vi "Conn Get Properties.vi"(4 "error in (no error)":errorcluster, 7 "connection reference":T2) -> (0 "error out":errorcluster, 1 "connection properties":T1, 3 "connection reference out":T2)   [LabVIEW 2017, in "NI_Database_API.lvlib"]
doc: "Gets properties of the object as determined by the inputs. This VI works for connections, commands, recordsets, columns, and parameters. Wire data to the reference input to determine the polymorphic instance to use or manually select the instance."
uses:
  <vilib>/addons/database/NI_Database_API.lvlib
  <vilib>/addons/database/Connection.llb/Conn ObjectReference.ctl
  <vilib>/addons/database/Connection.llb/Conn Properties.ctl
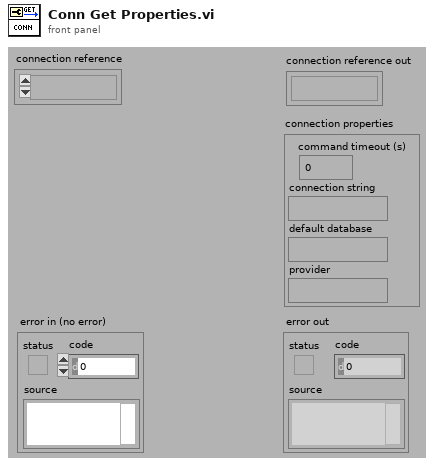
[diagram p1: front panel]
types:
  T1 = typedef "NI_Database_API.lvlib/Conn Properties.ctl" = cluster{"command timeout (s)":i32, "connection string":string, "default database":string, "provider":string}
  T2 = typedef "NI_Database_API.lvlib/Conn ObjectReference.ctl" = refnum<k1>
  T3 = typedef "NI_Database_API.lvlib/Conn DataMembers.ctl" = cluster{"ADODB._Connection":refnum<k7>, "recordset objects":i32, "command objects":i32}
  T4 = cluster{"CommandTimeout":i32, "ConnectionString":string, "DefaultDatabase":string, "Provider":string}
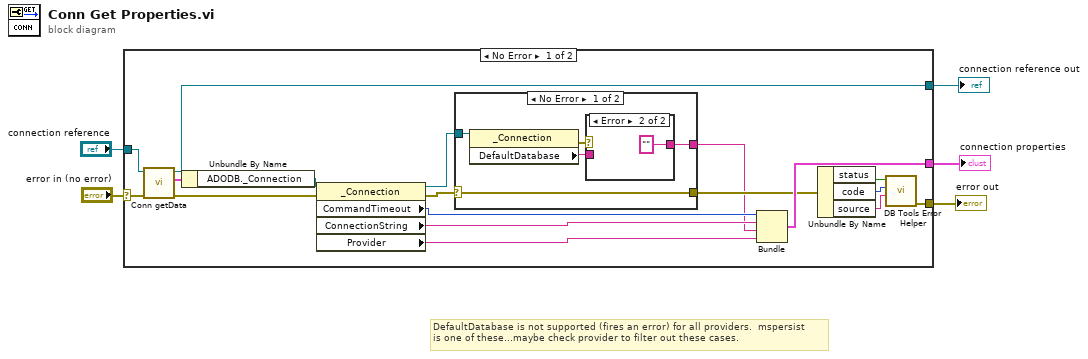
[diagram p0: block diagram]
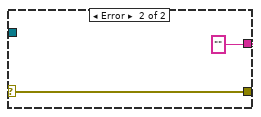
[diagram p3: hidden frame]
diagram:
  # "DefaultDatabase is not supported (fires an error) for all providers.  mspersist\nis one of these...maybe check provider to filter out these cases."
  n1 = case shown="No Error" "error in (no error)" {
    selector: "error in (no error)" -> [w11 w34]
    tunnel: "connection reference" -> [w23 w33]
    tunnel: [w20 _] -> w4
    tunnel: [w16 w33] -> w3
    tunnel: [w12 w34] -> w2
    frame No Error {
      n2 = call <vilib>:"Conn getData.vi"("error in (no error)"=w11, "connection reference"=w23) -> ("error out"=w18:errorcluster, "data"=w19:T3, "connection reference out"=w16:T2)  [unwired: 3 out]
      n3 = Unbundle By Name(w19) -> ("ADODB._Connection"=w17:refnum<k7>)
      n4 = property class="_Connection"(reference=w17, error in=w18) -> (reference out=w7:refnum<k7>, error out=w10:errorcluster, "CommandTimeout"=w22:i32, "ConnectionString"=w21:string, "Provider"=w9:string)
      n5 = case shown="No Error" w10 {
        selector: w10 -> [w24 w32]
        tunnel: [w24 w32] -> w8
        tunnel: w7 -> [w28 _]
        tunnel: [w25 ""] -> w6
        frame No Error {
          n6 = property class="_Connection"(reference=w28) -> (error out=w27:errorcluster, "DefaultDatabase"=w26:string)  [unwired: 1 in, 1 out]
          n7 = case shown="Error" w27 {
            tunnel: w26 -> [w29 _]
            tunnel: [w29 ""] -> w25
            frame No Error {
            }
            frame Error {
            }
          }
        }
        frame Error {
        }
      }
      n8 = Bundle("CommandTimeout"=w22, "ConnectionString"=w21, "DefaultDatabase"=w6, "Provider"=w9) -> (w20:T4)  [unwired: 1 out]
      n9 = Unbundle By Name(w8) -> ("status"=w14:bool, "code"=w13:i32, "source"=w15:string)
      n10 = call <vilib>:"DB Tools Error Helper.vi"("source"=w15, "code"=w13, "status"=w14) -> ("error out"=w12:errorcluster)  [unwired: 1 in, 7 out]
    }
    frame Error {
    }
  }
  "connection reference out" <- w3
  "error out" <- w2
  "connection properties" <- w4
